vi "TEST_Calibration.vi"() -> ()   [LabVIEW 2024]
panel:
  in  "Cal_Low_Laser_Reading":dbl=3.2789
  in  "Cal_High_Laser_Reading":dbl=4.132478
  in  "stop":bool
  in  "Boolean":bool
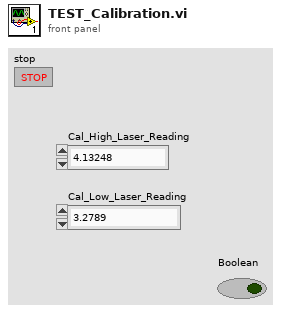
[diagram p1: front panel]
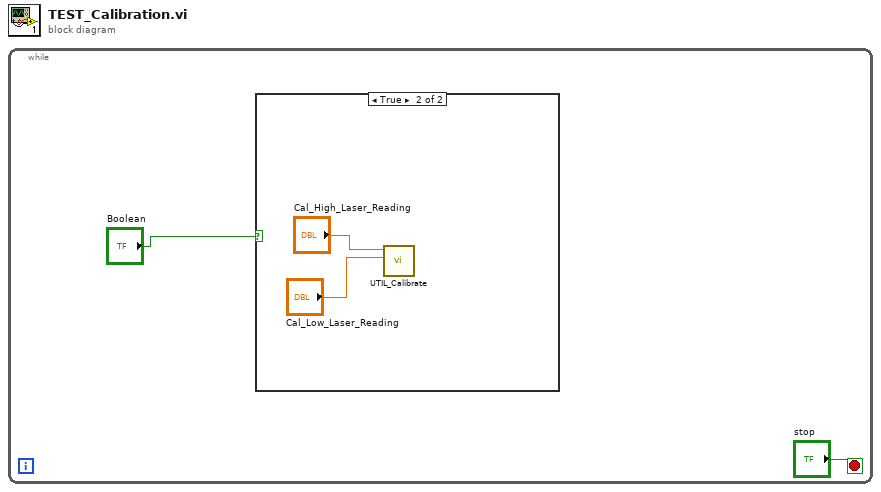
[diagram p0: block diagram]
diagram:
  n1 = while {
    stop <- "stop" stop-if-true
    n2 = case shown="True" "Boolean" {
      frame False {
      }
      frame True {
        n3 = call "UTIL_Calibrate.vi"("Cal_Low_Laser_Reading"="Cal_Low_Laser_Reading", "Cal_High_Laser_Reading"="Cal_High_Laser_Reading") -> ()  [unwired: 10 in]
      }
    }
  }
